vi "VciDeviceClose.vi"(3 "error in":errorcluster {"code" format="%.0x"}, 5 "Device Handle":u32) -> (0 "error out":errorcluster {"code" format="%.0x"})   [LabVIEW 2011]
doc: "Closes the VCI device specified by the device handle."
uses:
  vcilva.dll
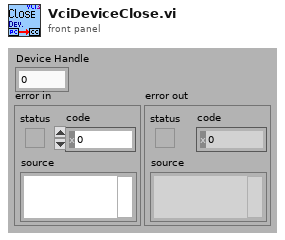
[diagram p1: front panel]
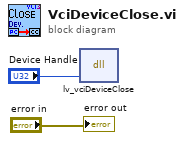
[diagram p0: block diagram]
diagram:
  n1 = dll-call lib="vcilva.dll" fn="lv_vciDeviceClose"("hDevice"="Device Handle") -> ()  [unwired: 5 in, 2 out]
  "error out" <- "error in"
